vi "Pole Placement Control Simulation.vi"() -> ()   [LabVIEW 2011]
uses:
  <vilib>/Simulation/Scripting/Companion Diagram/SimConfigNode/SimParams.ctl
  <vilib>/Simulation/Scripting/Companion Diagram/SimConfigNode/_simSolvers.ctl
  <vilib>/Simulation/Implementation/Shared/SIMSCR Execution Mode.ctl
  <vilib>/Platform/TimedLoop/XDataNode/timing_clust.ctl
  <vilib>/Platform/TimedLoop/XDataNode/nitl_modes.ctl
  <vilib>/Platform/TimedLoop/XDataNode/wakeup.ctl
  <vilib>/Simulation/Param Hierarchy/Typedefs/SIMPH Param Control Actions.ctl
  <vilib>/Simulation/Implementation/Shared/NILVSim_FinishedLate.vi
  <vilib>/Simulation/Utility/Implementation/SIM SimulationParams.vi
  <vilib>/Simulation/Utility/Implementation/SIM Halt.vi
  <vilib>/Simulation/Utility/Implementation/SIM Time.vi
  <vilib>/Simulation/SignalArithmetic/Implementation/NILVSim Gain.llb/SIM Gain (dot product).vi
  <vilib>/Simulation/DataSources/Implementation/NILVSim Signal Generator.llb/SIM Signal Generator (scalar).vi
  <vilib>/Simulation/SignalDisplay/Implementation/NILVSim Time Waveform.llb/SIM Time Waveform (scalar).vi
  <vilib>/Simulation/ContinuousLinear/Implementation/NILVSim State Space.llb/SIM State Space Distributor (SISO CD).vi
  <vilib>/Simulation/ContinuousLinear/Implementation/NILVSim State Space.llb/SIM State Space Collector (SISO CD).vi
  <vilib>/Simulation/Implementation/Shared/NILVSim_Manager.vi
  <vilib>/Simulation/Implementation/Shared/NILVSim_ParamChanged.vi
  <vilib>/Simulation/Implementation/Shared/NILVSim_FinalizeModel.vi
  <vilib>/Simulation/Utility/Implementation/NILVSim SimulationParams (core).vi
  <vilib>/Simulation/Utility/Implementation/NILVSim Get Time and IsAcceptedStep.vi
  <vilib>/imath/engines/lvmath2/RunTimeEngine/ErrorHandling/NIMS_Finalize Error.vi
  <vilib>/imath/engines/lvmath2/RunTimeEngine/Managers/WorkSpace/UID Generator.vi
  <vilib>/imath/engines/lvmath2/RunTimeEngine/NodeEndStatement/NIMS_NodeEndStatement_Get Vector.vi
  <instcachedir>/0/NIMS_NodeEndStatement_Get Vector_50E2F48DC826428EA11CD85545CBACBE.lvgen/NIMS_NodeEndStatement_Get Vector_50E2F48DC826428EA11CD85545CBACBE_001.vi
  <vilib>/imath/engines/lvmath/Functions/Error Handling/MergeErrorsWrapper.vi
  <vilib>/imath/engines/lvmath2/RunTimeEngine/Managers/SymbolTable/Clear UID.vi
  <vilib>/imath/engines/lvmath2/RunTimeEngine/NodeEndStatement/NIMS_NodeEndStatement_Output.vi
  <instcachedir>/0/NIMS_NodeEndStatement_Output_53EC0D466D134D7ABD903AC30B43404B.lvgen/NIMS_NodeEndStatement_Output_53EC0D466D134D7ABD903AC30B43404B_005.vi
  <instcachedir>/0/NIMS_NodeEndStatement_Output_53EC0D466D134D7ABD903AC30B43404B.lvgen/NIMS_NodeEndStatement_Output_53EC0D466D134D7ABD903AC30B43404B_010.vi
  <vilib>/imath/engines/lvmath2/RunTimeEngine/RunTimeType/NIMS_RunTimeType_From StrictType (excl LVString).vi
  <instcachedir>/0/NIMS_RunTimeType_From StrictType (excl LVString)_46AE8B54A11948F0BCCEB8091EE7AA4C.lvgen/NIMS_RunTimeType_From StrictType (excl LVString)_46AE8B54A11948F0BCCEB8091EE7AA4C_000.vi
  <vilib>/imath/engines/lvmath2/RunTimeEngine/LocalVariableDefStatement/MC_LocalVariableDefStatement_Display.vi
  <vilib>/imath/engines/lvmath/Plug In/Control Design/BuiltInFunctions/ss/NIMS_CD_ss(A,B,C,D).vi
  <instcachedir>/0/NIMS_RunTimeType_From StrictType (excl LVString)_46AE8B54A11948F0BCCEB8091EE7AA4C.lvgen/NIMS_RunTimeType_From StrictType (excl LVString)_46AE8B54A11948F0BCCEB8091EE7AA4C_028.vi
  <vilib>/imath/engines/lvmath/Plug In/Control Design/BuiltInFunctions/poleplace/NIMS_CD_poleplace(A,B,poles,STR).vi
  <vilib>/Simulation/Implementation/Shared/SIM Unbundle Sim Info.vi
  <vilib>/Simulation/Implementation/Shared/NILVSim_GetModelError.vi
  <vilib>/Simulation/Implementation/Shared/SIM Bundle Sim Info.vi
  <vilib>/Simulation/Implementation/Shared/NILVSim_Initialize.vi
  <vilib>/Simulation/Scripting/Companion Diagram/SimConfigNode/SimDog.xnode
  <vilib>/addons/Control Design/_Model Construction/Model Typedefs.llb/CD State Space Model (MIMO).ctl
  <vilib>/addons/Control Design/_Model Construction/Model Typedefs.llb/CD General Elements.ctl
  <vilib>/Platform/TimedLoop/XDataNode/XDataNode.xnode
  <vilib>/Simulation/Implementation/XNodeFramework/SimXNode/SimX.xnode
  <vilib>/addons/Control Design/_Model Construction/NI_LinSys_Model Typedefs.lvlib
  <vilib>/imath/engines/lvmath2/RunTimeEngine/Managers/SymbolTable/NIMS_WorkSpace.lvlib
  <vilib>/Simulation/ContinuousLinear/Implementation/NILVSim State Space.llb/SIM State Space (SISO CD).vi
  <vilib>/Platform/TimedLoop/XDataNode/XDNodeRunTimeDep.lvlib
  <vilib>/Simulation/Implementation/Shared/NI_SIM_Implementation.lvlib
panel:
  out "Waveform Chart":waveform(dbl)(graph)
  in  "amplitude (rad)":dbl(slide)=0.52 scale=0.0..3.0
  in  "frequency (Hz)":dbl(slide)=0.4 scale=0.0..10.0
  out "simulation time":dbl=18.68
  in  "stop":bool
  out "Finished Late?":bool
  # "Pulse Train Input"
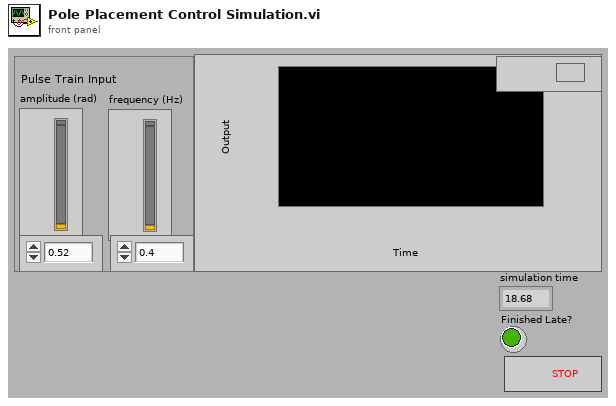
[diagram p1: front panel]
types:
  T1 = typedef "NI_LinSys_Model Typedefs.lvlib/CD State Space Model (MIMO).ctl" = cluster{"properties":T2, "A":dbl[][], "B":dbl[][], "C":dbl[][], "D":dbl[][], "StateNames":string[], "Transport Delay":dbl[][]}
  T2 = typedef "NI_LinSys_Model Typedefs.lvlib/CD General Elements.ctl" = cluster{"Model name":string, "Input names":string[], "Output names":string[], "Input Delays":dbl[], "Output Delays":dbl[], "Sampling Time":dbl, "Notes":string}
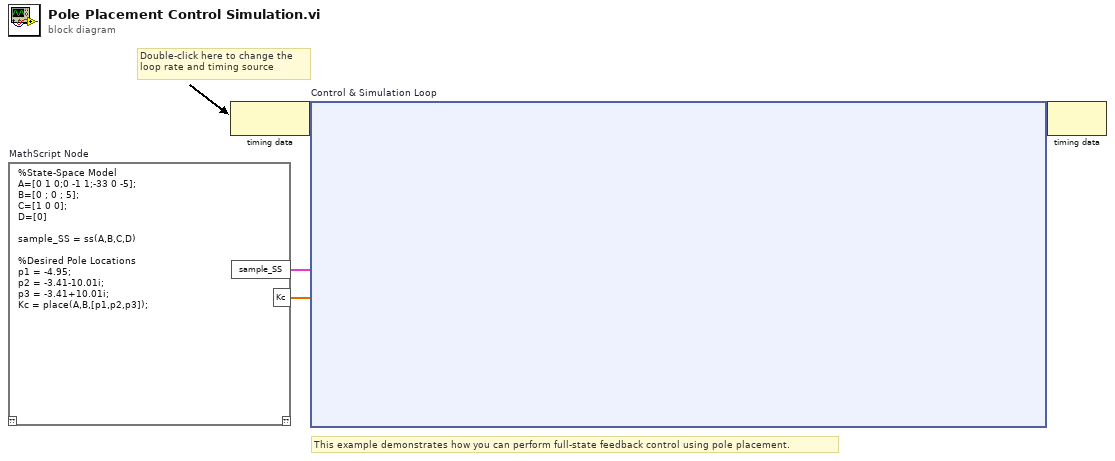
[diagram p0: block diagram]
diagram:
  # "This example demonstrates how you can perform full-state feedback control using pole placement."
  # "Double-click here to change the\nloop rate and timing source"
  n1 = mathscript code="%State-Space Model\nA=[0 1 0;0 -1 1;-33 0 -5];\nB=[0 ; 0 ; 5];\nC=[1 0 0];\nD=[0]\n\nsample_SS = ss(A,B,C,D)\n\n%Desired Pole Locations\np1 = -4.95;\np2 = -3.41-10.01i;\np3 = -3.41+10.01i;\nKc = place(A,B,[p1,p2,p3]);"() -> ("sample_SS"=w2:T1, "Kc"=w1:dbl[])  [unwired: 1 in, 1 out]
  n2 = node-c288() -> (w4:variant)  [unwired: 1 in]
  n3 = node-c254 "Control & Simulation Loop"(w4, w2, w1) -> (w3:variant)
  n4 = node-c288(w3) -> ()  [unwired: 1 out]
